vi "dfd_NPR Cosine-Modulated Prototype Filter Design Iteration.vi"(6 "gama":dbl, 7 "number of bands":i32, 8 "error in (no error)":errorcluster, 9 "order":i32, 10 "Us":dbl[][](array[numeric]), 11 "half initial h":dbl[](array[numeric])) -> (0 "error out":errorcluster, 3 "half h":dbl[](array[numeric]))   [LabVIEW 2017, in "NI_DigFilter_FilterBank.lvlib"]
uses:
  <vilib>/addons/Digital Filter Design/NI_DigFilter_FilterBank.lvlib
  <vilib>/Analysis/baseanly.llb/Real A x B.vi
  <vilib>/Analysis/baseanly.llb/A x Vector.vi
  <vilib>/addons/Digital Filter Design/_Misc.llb/dfd_Error Cluster From Error Code (Array).vi
  <vilib>/addons/Digital Filter Design/_Misc.llb/dfd_X Equal Y (Array).vi
  <vilib>/Analysis/baseanly.llb/Real Inverse Matrix.vi
  <vilib>/Analysis/Matrix/Numeric/Add/Add - RM,RM.vi
  <vilib>/Analysis/NI_AALBase.lvlib
  <vilib>/addons/Digital Filter Design/NI_DigFilterLicensed.lvlib
  <vilib>/Analysis/Matrix/NI_Matrix.lvlib
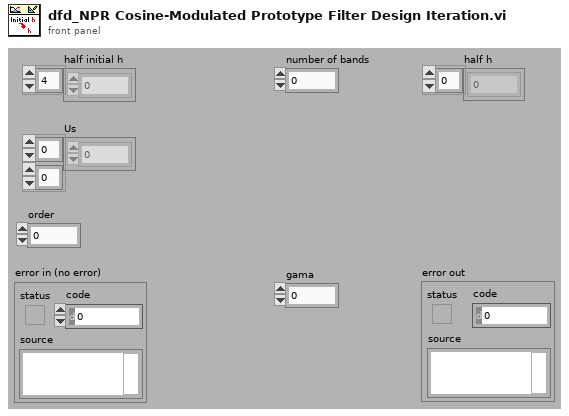
[diagram p1: front panel]
types:
  T1 = enum32{"General", "Positive Definite", "Lower Triangular", "Upper Triangular"}
  T2 = typedef "NI_Matrix.lvlib/RealMatrix.ctl" = dbl[][]
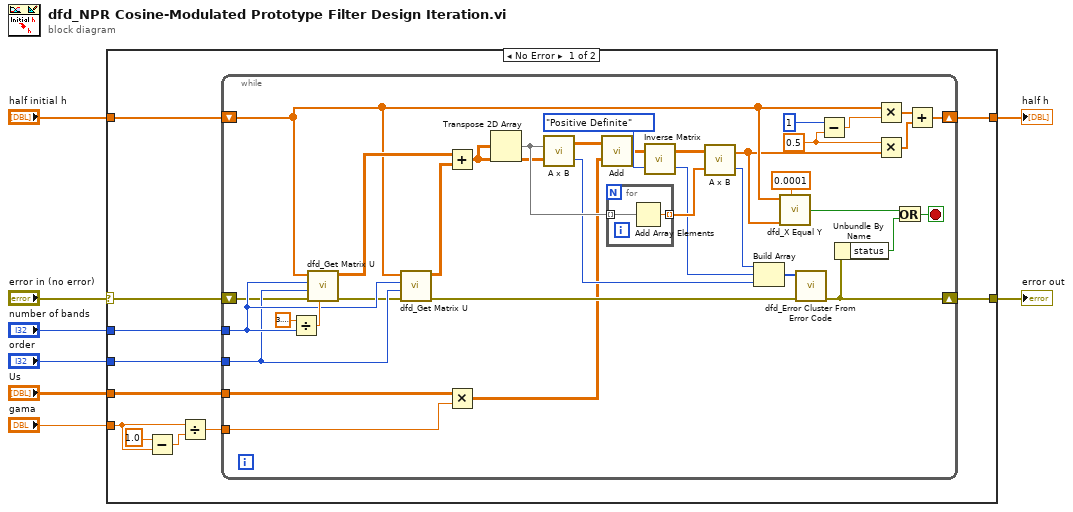
[diagram p0: block diagram]
diagram:
  n1 = case shown="No Error" "error in (no error)" {
    selector: "error in (no error)" -> [w9 w58]
    tunnel: [w19 _] -> w8
    tunnel: "order" -> [w18 _]
    tunnel: "number of bands" -> [w17 _]
    tunnel: "Us" -> [w16 _]
    tunnel: "half initial h" -> [w15 _]
    tunnel: [w14 w58] -> w3
    tunnel: "gama" -> [w11 _]
    frame No Error {
      n2 = Subtract(x=1.0, y=w11) -> (x-y=w13:dbl)
      n3 = Divide(x=w11, y=w13) -> (x/y=w10:dbl)
      n4 = while {
        tunnel: w17 -> [w40]
        tunnel: w18 -> [w39]
        shift-right: [w47] -> w19
        shift-left: w15 -> [w25]
        tunnel: w16 -> [w30]
        shift-right: [w23] -> w14
        shift-left: w9 -> [w38]
        tunnel: w10 -> [w28]
        stop <- w20 stop-if-true
        w42 = 0.5 ("gama")
        n5 = Divide(x=3.141592653589793, y=w40) -> (x/y=w46:dbl)
        n6 = call <vilib>:"dfd_Get Matrix U.vi"("para"=w46, "error in (no error)"=w38, "order"=w39, "number of bans"=w40, "half h"=w25) -> ("error out"=w37:errorcluster, "U"=w26:dbl[][])  [unwired: 5 in]
        n7 = call <vilib>:"dfd_Get Matrix U.vi"("error in (no error)"=w37, "order"=w39, "number of bans"=w40, "half h"=w25) -> ("error out"=w36:errorcluster, "U"=w27:dbl[][])  [unwired: 6 in]
        n8 = Add(x=w26, y=w27) -> (x+y=w29:dbl[][])
        n9 = Multiply(x=w30, y=w28) -> (x*y=w31:dbl[][])
        n10 = Transpose 2D Array(2D array=w29) -> (transposed array=w55:dbl[][])
        n11 = call-poly <vilib>:"A x B.vi"("B"=w29, "A"=w55) -> ("error"=w35:i32, "A x B"=w41:T2)
        n12 = call-poly <vilib>:"Add.vi"("Real Matrix B"=w31, "Real Matrix A"=w41) -> ("A + B"=w44:T2)
        n13 = for {
          tunnel: w55 -> [w57] mode=indexing
          tunnel: [w56] -> w53 mode=indexing
          n14 = Add Array Elements(numeric array=w57) -> (sum=w56:dbl)
        }
        n15 = call-poly <vilib>:"Inverse Matrix.vi"("matrix type"=T1."Positive Definite", "Input Matrix"=w44) -> ("error"=w34:i32, "Inverse Matrix"=w54:T2)
        n16 = call-poly <vilib>:"A x B.vi"("Vector"=w53, "A"=w54) -> ("error"=w33:i32, "A x Vector"=w24:dbl[])
        n17 = Build Array(w33, w34, w35) -> (w32:i32[])
        n18 = call-poly <vilib>:"dfd_X Equal Y.vi"("x"=w25, "y"=w24, "esp"=0.0001) -> ("x = y?"=w22:bool)  [unwired: 4 in]
        n19 = call-poly <vilib>:"dfd_Error Cluster From Error Code.vi"("error in (no error)"=w36, "error code (0)"=w32) -> ("error out"=w23:errorcluster)  [unwired: 9 in]
        n20 = Subtract(x=1, y=w42) -> (x-y=w51:dbl)
        n21 = Unbundle By Name(w23) -> ("status"=w21:bool)
        n22 = Multiply(x=w25, y=w51) -> (x*y=w50:dbl[])
        n23 = Multiply(x=w42, y=w24) -> (x*y=w49:dbl[])
        n24 = Or(x=w22, y=w21) -> (x .or. y?=w20:bool)
        n25 = Add(x=w50, y=w49) -> (x+y=w47:dbl[])
      }
    }
    frame Error {
    }
  }
  "half h" <- w8
  "error out" <- w3
